vi "Weather_Station_Model.vi"() -> (1 "Supported?":bool, 2 "Weather station model":string)   [LabVIEW 2013]
uses:
  VantagePro.dll
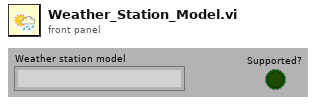
[diagram p1: front panel]
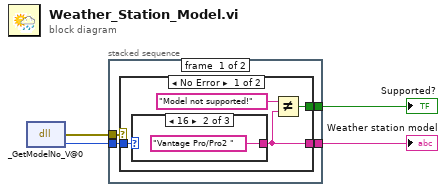
[diagram p0: block diagram]
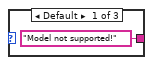
[diagram p2: hidden frame]
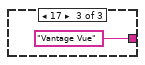
[diagram p3: hidden frame]
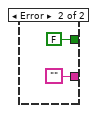
[diagram p4: hidden frame]
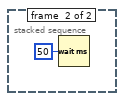
[diagram p5: hidden frame]
diagram:
  n1 = dll-call lib="C:/Users/Bob van Eijk/Desktop/LabView Projects 13/HiSPARC Weather Station/Develop/VantagePro.dll" fn="_GetModelNo_V@0" label="Call Library Function\nGetModelNo"() -> (error out=w1:errorcluster, "return type"=w4:i16)  [unwired: 3 in, 1 out]
  n2 = stacked-sequence {
    tunnel: w4 -> [w8 _]
    tunnel: [w7 _] -> w3
    tunnel: [w6 _] -> w2
    tunnel: w1 -> [w5 _]
    frame #0 {
      n3 = case shown="No Error" w5 {
        tunnel: w8 -> [w12 _]
        tunnel: [w10 ""] -> w7
        tunnel: [w9 FALSE] -> w6
        frame No Error {
          n4 = case shown="16" w12 {
            tunnel: ["Model not supported!" "Vantage Pro/Pro2 " "Vantage Vue"] -> w10
            frame Default {
            }
            frame 16 {
            }
            frame 17 {
            }
          }
          n5 = Not Equal?(x="Model not supported!", y=w10) -> (x != y?=w9:bool)
        }
        frame Error {
        }
      }
    }
    frame #1 {
      n6 = Wait (ms)(milliseconds to wait=u32 50) -> ()  [unwired: 1 out]
    }
  }
  "Weather station model" <- w3
  "Supported?" <- w2
